vi "saveGenerateName.vi"(9 "use default folder":bool=TRUE, 10 "Type":u16(ring) items=["mic", "pd", "processed", "crd", "sweeps", "compiled"], 11 "working directory":path) -> (2 "file path":path, 3 "working directory":path)   [LabVIEW 2011]
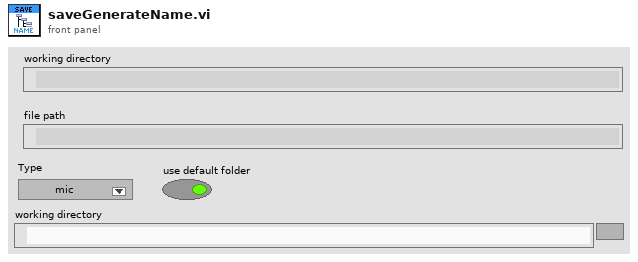
[diagram p1: front panel]
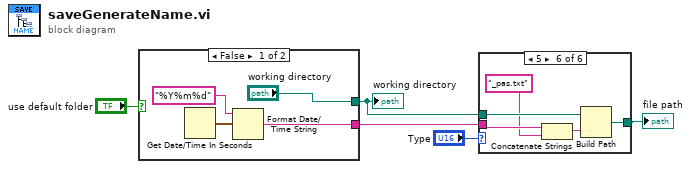
[diagram p0: block diagram]
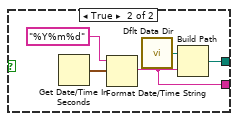
[diagram p2: hidden frame]
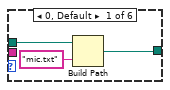
[diagram p3: hidden frame]
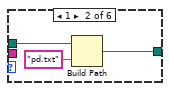
[diagram p4: hidden frame]
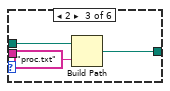
[diagram p5: hidden frame]
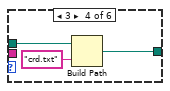
[diagram p6: hidden frame]
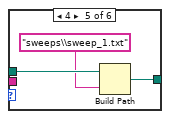
[diagram p7: hidden frame]
diagram:
  n1 = case shown="False" "use default folder" {
    tunnel: ["working directory" w14] -> w4
    tunnel: [w6 w10] -> w1
    frame False {
      n2 = Get Date/Time In Seconds() -> (seconds since 1Jan1904=w7:timestamp)
      n3 = Format Date/Time String(time format string (%c)="%Y%m%d", seconds (now)=w7) -> (date/time string=w6:string)  [unwired: 1 in]
    }
    frame True {
      n4 = Get Date/Time In Seconds() -> (seconds since 1Jan1904=w12:timestamp)
      n5 = Format Date/Time String(time format string (%c)="%Y%m%d", seconds (now)=w12) -> (date/time string=w10:string)  [unwired: 1 in]
      n6 = call <vilib>:"Dflt Data Dir.vi"() -> ("App:Default Data Directory"=w11:path)
      n7 = Build Path(base path=w11, name or relative path=w10) -> (appended path=w14:path)
    }
  }
  "working directory" <- w4
  n8 = case shown="5" "Type" {
    tunnel: w4 -> [w15 w20 w23 w26 w29 w34]
    tunnel: [w16 w18 w21 w24 w27 w33] -> w5
    tunnel: w1 -> [_ _ _ _ _ w31]
    frame 0, Default {
      n9 = Build Path(base path=w15, name or relative path="mic.txt") -> (appended path=w16:path)
    }
    frame 1 {
      n10 = Build Path(base path=w20, name or relative path="pd.txt") -> (appended path=w18:path)
    }
    frame 2 {
      n11 = Build Path(base path=w23, name or relative path="proc.txt") -> (appended path=w21:path)
    }
    frame 3 {
      n12 = Build Path(base path=w26, name or relative path="crd.txt") -> (appended path=w24:path)
    }
    frame 4 {
      n13 = Build Path(base path=w29, name or relative path="sweeps\\sweep_1.txt") -> (appended path=w27:path)
    }
    frame 5 {
      n14 = Concatenate Strings(w31, "_pas.txt" ("name or relative path")) -> (w32:string)
      n15 = Build Path(base path=w34, name or relative path=w32) -> (appended path=w33:path)
    }
  }
  "file path" <- w5
